vi "Add Folder to Target.vi"(8 "error in (no error)":errorcluster, 9 "Name":string="Descriptor", 10 "Target Name":string="My Computer", 11 "Project Sync Tools in":refnum<class "Project Sync Tools.lvclass">) -> (0 "error out":errorcluster, 2 "Folder Item ref":refnum<vi>, 3 "Project Sync Tools out":refnum<class "Project Sync Tools.lvclass">)   [LabVIEW 2019, in "Project Sync Tools.lvclass"]
uses:
  Project Sync Tools.lvclass
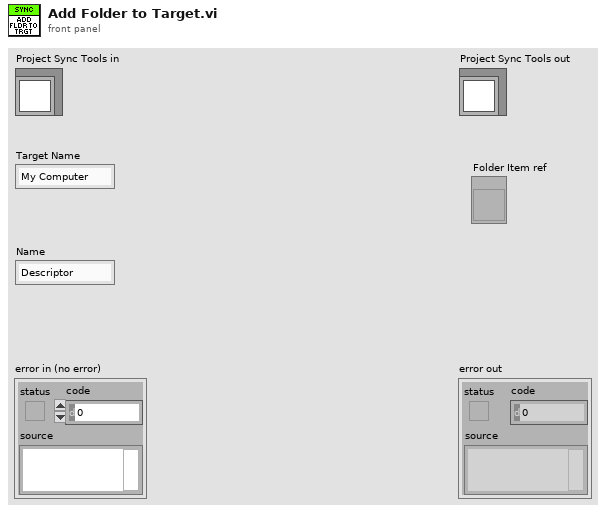
[diagram p1: front panel]
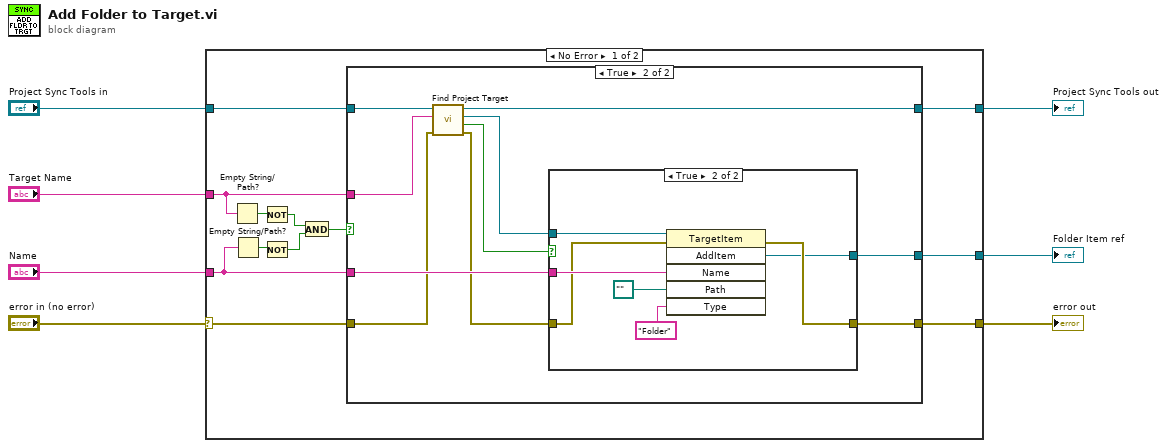
[diagram p0: block diagram]
diagram:
  n1 = case shown="No Error" "error in (no error)" {
    selector: "error in (no error)" -> [w15 w41]
    tunnel: [w17 w41] -> w6
    tunnel: [w18 w40] -> w4
    tunnel: "Project Sync Tools in" -> [w19 w40]
    tunnel: "Target Name" -> [w12 _]
    tunnel: "Name" -> [w11 _]
    tunnel: [w16 _] -> w3
    frame No Error {
      n2 = Empty String/Path?(string/path=w12) -> (empty?=w13:bool)
      n3 = Empty String/Path?(string/path=w11) -> (empty?=w14:bool)
      n4 = Not(x=w13) -> (.not. x?=w10:bool)
      n5 = Not(x=w14) -> (.not. x?=w9:bool)
      n6 = And(x=w10, y=w9) -> (x .and. y?=w8:bool)
      n7 = case shown="True" w8 {
        tunnel: w19 -> [w21 w30]
        tunnel: [w21 w29] -> w18
        tunnel: w12 -> [_ w28]
        tunnel: w11 -> [_ w27]
        tunnel: [w20 w26] -> w17
        tunnel: [_ w25] -> w16
        tunnel: w15 -> [w20 w23]
        frame False {
        }
        frame True {
          n8 = call "Find Project Target.vi"("error in (no error)"=w23, "Target Name"=w28, "Project Sync Tools in"=w30) -> ("error out"=w22:errorcluster, "Found ?"=w24:bool, "TargetItem out"=w31:refnum<vi>, "Project Sync Tools out"=w29:refnum<class "Project Sync Tools.lvclass">)  [unwired: 5 in]
          n9 = case shown="True" w24 {
            tunnel: w31 -> [_ w37]
            tunnel: w27 -> [_ w36]
            tunnel: w22 -> [w32 w35]
            tunnel: [w32 w34] -> w26
            tunnel: [_ w33] -> w25
            frame False {
            }
            frame True {
              n10 = invoke class="TargetItem" method="AddItem"(reference=w37, error in=w35, "Name"=w36, "Path"=path "", "Type"="Folder") -> (error out=w34:errorcluster, "AddItem"=w33:refnum<vi>)  [unwired: 1 in, 4 out]
            }
          }
        }
      }
    }
    frame Error {
    }
  }
  "error out" <- w6
  "Project Sync Tools out" <- w4
  "Folder Item ref" <- w3
